vi "Configure Clocks.vi"(0 "Register Bus":T1, 1 "scope":string(combo)="rx", 5 "clock source":string(combo)="Internal" caption="Clock Source", 7 "reference clock source":string(combo)="PXI_CLK" caption="Reference Clock Source", 11 "error in":errorcluster) -> (4 "Register Bus (out)":T1, 15 "error out":errorcluster)   [LabVIEW 2017]
doc: "Configure the device's clocks based on the clock source and the reference clock source.\n\n<B>Input Parameters</B>\n\n<B>Register Bus</B> The Register Bus object created by the ni579x Open VI and used as the session handle for the NI-579x Configuration Design Library.\n\n<B>scope</B> is the channel to configure clocks for. The options are \"rx\" and \"tx\".\n\n<B>clock source</B> is the source of the Sample Clock. Can be \"Internal\" or the \"ClkIn\" front-panel terminal.\n\n<B>reference clock source</B> is the source of the clock that serves as a reference clock for the sample clock and local oscillator. Can be \"Internal\", \"PXI_CLK\" for the PXI backplane reference (sync clock), or \"ClkIn\" for the front-panel terminal.\n\n<B>error in</B> describes error conditions that occur before this node runs. This input provides standard 'error in' functionality.\n\n<B>Output Parameters</B>\n\n<B>Register Bus (out)</B> The Register Bus object created by the ni579x Open VI and used as the session handle for the NI-579x Configuration Design Library.\n\n<B>error out</B> contains error information. This output provides standard 'error out' functionality."
uses:
  <instrlib>/_niInstr/Register Bus/v0/Host/Public/Register Bus Session.ctl
  <instrlib>/_niInstr/Register Bus/v0/Host/Private/Session Data.ctl
  <instrlib>/ni579x/Config/v2/Host/ni579x Config v2 Host.lvlib
  <instrlib>/_niInstr/Register Bus/v0/Host/niInstr Register Bus v0 Host.lvlib
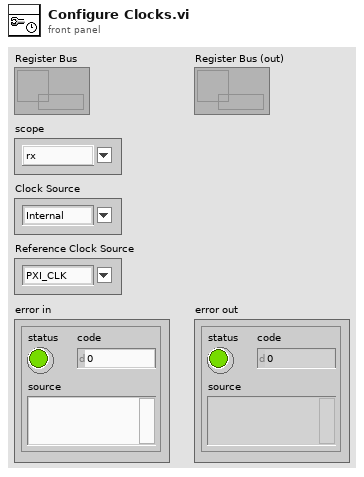
[diagram p1: front panel]
types:
  T1 = typedef "niInstr Register Bus v0 Host.lvlib/Register Bus Session.ctl" = refnum<queue>
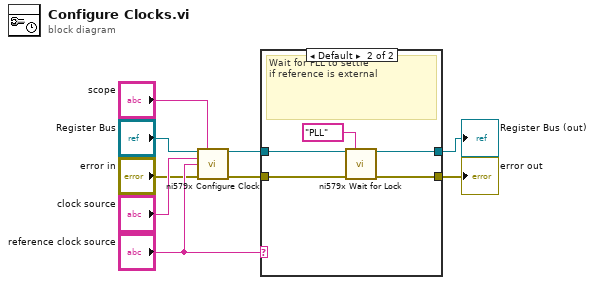
[diagram p0: block diagram]
diagram:
  n1 = call <instrlib>:"ni579x Configure Clock.vi"("Register Bus"="Register Bus", "scope"="scope", "clock source"="clock source", "reference clock source"="reference clock source", "Error In"="error in") -> ("Register Bus (out)"=w5:T1, "Error Out"=w4:errorcluster)  [unwired: 9 in]
  n2 = case shown="Default" "reference clock source" {
    tunnel: w4 -> [w10 w16]
    tunnel: w5 -> [w11 w15]
    tunnel: [w11 w14] -> w7
    tunnel: [w10 w13] -> w3
    frame "Internal" {
      # "When using an internal reference clock, there's no need to wait for the PLL to lock."
    }
    frame Default {
      # "Wait for PLL to settle\nif reference is external"
      n3 = call <instrlib>:"ni579x Wait for Lock.vi"("Register Bus"=w15, "scope"="PLL", "Error In"=w16) -> ("Register Bus (out)"=w14:T1, "Error Out"=w13:errorcluster)  [unwired: 11 in]
    }
  }
  "Register Bus (out)" <- w7
  "error out" <- w3
